vi "avion.vi"() -> ()   [LabVIEW 2012]
panel:
  out "Clase Reservada":string
  out "Avion lleno Clase Economica":bool
  out "Avion lleno Primera clase":bool
  out "Numero de Asientos":dbl
  in  "Presione OK para Seleccionar":bool
  in  "Escoja la clase de asientos":u16(ring) items=["Primera Clase", "Clase Economica"]
  out "Asientos de Pasajeros":dbl[](array[numeric])
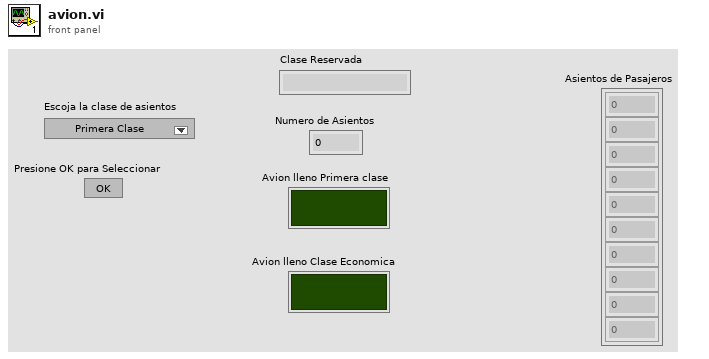
[diagram p1: front panel]
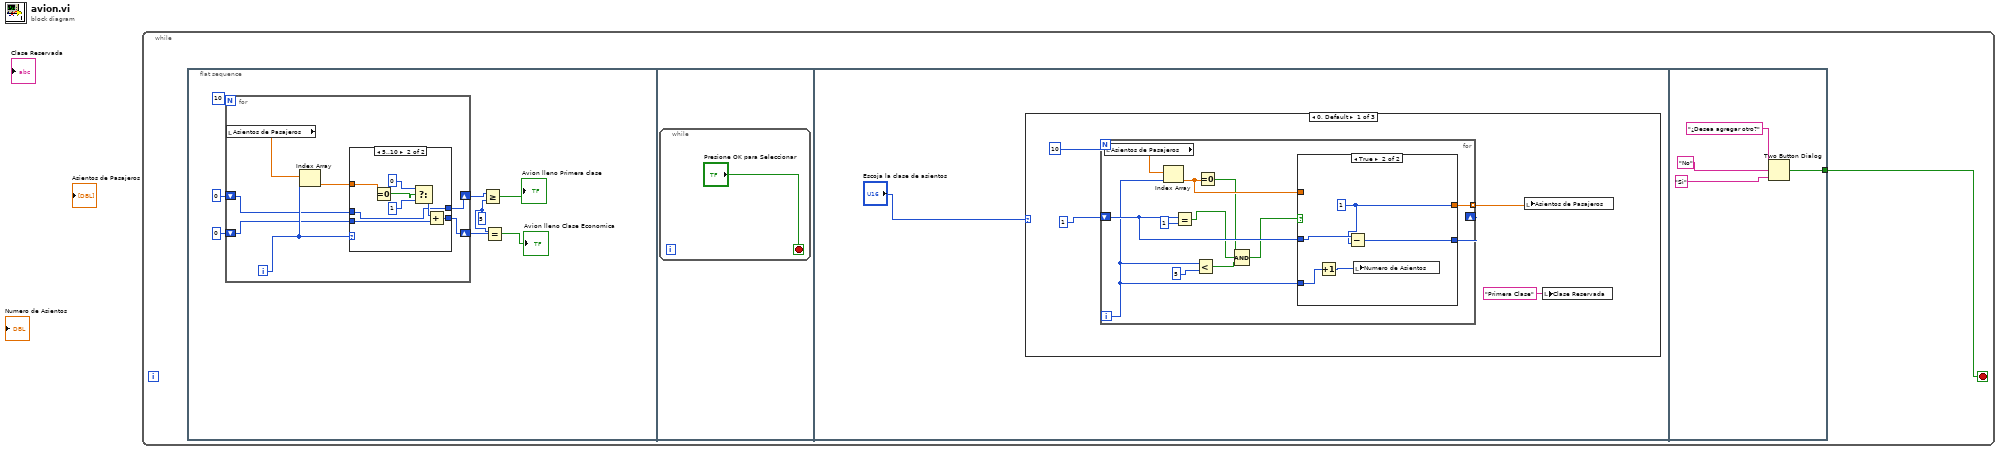
[diagram p0: block diagram]
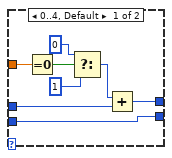
[diagram p2: hidden frame]
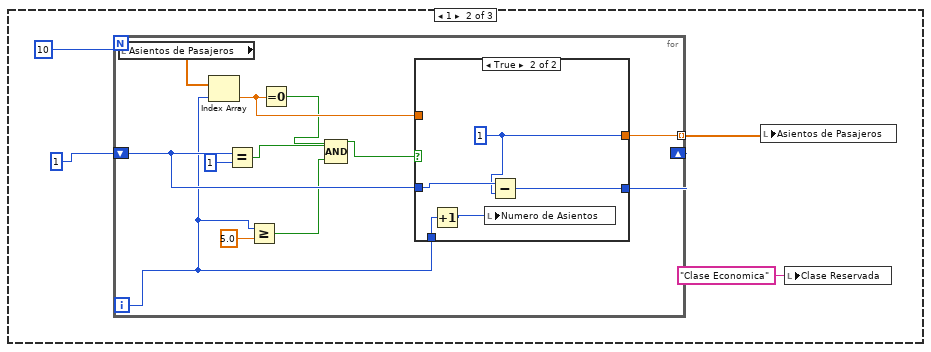
[diagram p4: hidden frame]
diagram:
  n1 = while {
    stop <- w1 stop-if-true
    n2 = flat-sequence {
      tunnel: [w81] -> w1
      frame #0 {
        w3 = 5
        n3 = for {
          N: 10 -> [_]
          shift-right: [w13] -> w2
          shift-left: 0 -> [w11]
          shift-right: [w12] -> w6
          shift-left: 0 -> [w10]
          i -> [w15]
          n4 = local read "Asientos de Pasajeros"() -> (w16:dbl[])
          n5 = Index Array(array=w16, index=w15) -> (element=w14:dbl)
          n6 = case shown="5..10" w15 {
            tunnel: w14 -> [w24 w32]
            tunnel: [w20 w25] -> w13
            tunnel: w11 -> [w19 w25]
            tunnel: [w17 w31] -> w12
            tunnel: w10 -> [w17 w27]
            frame 0..4, Default {
              n7 = Equal To 0?(x=w24) -> (x = 0?=w23:bool)
              n8 = Select(t=0, s=w23, f=1) -> (s? t:f=w21:i32)
              n9 = Add(x=w21, y=w19) -> (x+y=w20:i32)
            }
            frame 5..10 {
              n10 = Equal To 0?(x=w32) -> (x = 0?=w29:bool)
              n11 = Select(t=0, s=w29, f=1) -> (s? t:f=w28:i32)
              n12 = Add(x=w28, y=w27) -> (x+y=w31:i32)
            }
          }
        }
        n13 = Greater Or Equal?(x=w2, y=w3) -> (x >= y?=→"Avion lleno Primera clase":bool)
        n14 = Equal?(x=w3, y=w6) -> (x = y?=→"Avion lleno Clase Economica":bool)
      }
      frame #1 {
        n15 = while {
          stop <- "Presione OK para Seleccionar" stop-if-true
        }
      }
      frame #2 {
        n16 = case shown="0, Default" "Escoja la clase de asientos" {
          frame 0, Default {
            n17 = for {
              N: 10 -> [_]
              shift-right: [w45] -> _
              shift-left: 1 -> [w48]
              tunnel: [w47] -> w36 mode=indexing
              i -> [w39]
              n18 = local read "Asientos de Pasajeros"() -> (w50:dbl[])
              n19 = Index Array(array=w50, index=w39) -> (element=w46:dbl)
              n20 = Equal?(x=w48, y=1) -> (x = y?=w43:bool)
              n21 = Less?(x=w39, y=5) -> (x < y?=w42:bool)
              n22 = Equal To 0?(x=w46) -> (x = 0?=w44:bool)
              n23 = Compound Arithmetic op=AND(w44, w43, w42) -> (w41:bool)
              n24 = case shown="True" w41 {
                tunnel: w48 -> [w51 w57]
                tunnel: [w52 w56] -> w47
                tunnel: w46 -> [w52 _]
                tunnel: [w51 w55] -> w45
                tunnel: w39 -> [_ w54]
                frame False {
                }
                frame True {
                  w56 = 1
                  n25 = Increment(x=w54) -> (x+1=w53:i32)
                  n26 = Subtract(x=w57, y=w56) -> (x-y=w55:i32)
                  n27 = local write "Numero de Asientos"(w53) -> ()
                }
              }
            }
            n28 = local write "Asientos de Pasajeros"(w36) -> ()
            n29 = local write "Clase Reservada"("Primera Clase" ("Clase Reservada")) -> ()
          }
          frame 1 {
            n30 = for {
              N: 10 -> [_]
              shift-right: [w68] -> _
              shift-left: 1 -> [w71]
              tunnel: [w70] -> w59 mode=indexing
              i -> [w62]
              n31 = local read "Asientos de Pasajeros"() -> (w73:dbl[])
              n32 = Index Array(array=w73, index=w62) -> (element=w69:dbl)
              n33 = Equal?(x=w71, y=1) -> (x = y?=w66:bool)
              n34 = Greater Or Equal?(x=w62, y=5.0) -> (x >= y?=w63:bool)
              n35 = Equal To 0?(x=w69) -> (x = 0?=w67:bool)
              n36 = Compound Arithmetic op=AND(w67, w66, w63) -> (w65:bool)
              n37 = case shown="True" w65 {
                tunnel: w71 -> [w74 w80]
                tunnel: [w75 w79] -> w70
                tunnel: w69 -> [w75 _]
                tunnel: [w74 w78] -> w68
                tunnel: w62 -> [_ w76]
                frame False {
                }
                frame True {
                  w79 = 1
                  n38 = Increment(x=w76) -> (x+1=w77:i32)
                  n39 = local write "Numero de Asientos"(w77) -> ()
                  n40 = Subtract(x=w80, y=w79) -> (x-y=w78:i32)
                }
              }
            }
            n41 = local write "Asientos de Pasajeros"(w59) -> ()
            n42 = local write "Clase Reservada"("Clase Economica" ("Clase Reservada")) -> ()
          }
          frame 2 {
          }
        }
      }
      frame #3 {
        n43 = Two Button Dialog(message="¿Desea agregar otro?", 1:"Si", 2:"No") -> (T button?=w81:bool)
      }
    }
  }
